vi "Get Active ProjectPath.vi"(11 "error in (no error)":errorcluster) -> (4 "Project Path":path, 15 "error out":errorcluster)   [LabVIEW 2021, in "Measurement Builder.lvlib"]
uses:
  Measurement Builder.lvlib
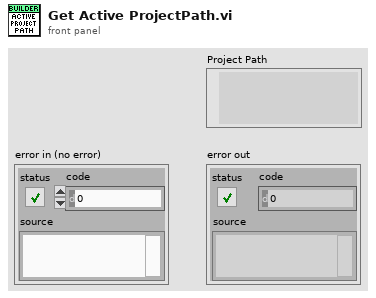
[diagram p1: front panel]
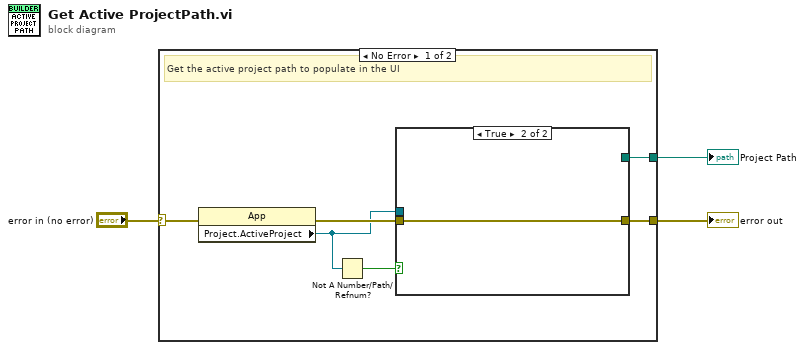
[diagram p0: block diagram]
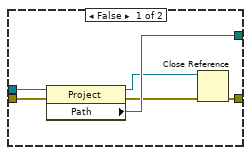
[diagram p2: hidden frame]
diagram:
  n1 = case shown="No Error" "error in (no error)" {
    selector: "error in (no error)" -> [w9 w17]
    tunnel: [w7 _] -> w2
    tunnel: [w6 w17] -> w1
    frame No Error {
      # "Get the active project path to populate in the UI"
      n2 = property class="App"(error in=w9) -> (error out=w8:errorcluster, "Project.ActiveProject"=w5:refnum<vi>)  [unwired: 1 in, 1 out]
      n3 = Not A Number/Path/Refnum?(number/path/refnum=w5) -> (NaN/Path/Refnum?=w4:bool)
      n4 = case shown="True" w4 {
        tunnel: w8 -> [w15 w16]
        tunnel: [w14 _] -> w7
        tunnel: [w11 w16] -> w6
        tunnel: w5 -> [w10 _]
        frame False {
          n5 = property class="Project"(reference=w10, error in=w15) -> (reference out=w12:refnum<vi>, error out=w13:errorcluster, "Path"=w14:path)
          n6 = Close Reference(reference=w12, error in (no error)=w13) -> (error out=w11:errorcluster)
        }
        frame True {
        }
      }
    }
    frame Error {
    }
  }
  "error out" <- w1
  "Project Path" <- w2
